vi "solar_voy_def Export (Mods_Limits).vi"(10 "CMD":enum8{"CMD", "TLM"}(ring), 11 "LIMITS":T1) -> (3 "LIMITS_DEF":string)   [LabVIEW 2018]
doc: "This exports a COSMOS limits modifier to string."
uses:
  solar_voy_def_ctl MODIFIERS LIMITS.ctl
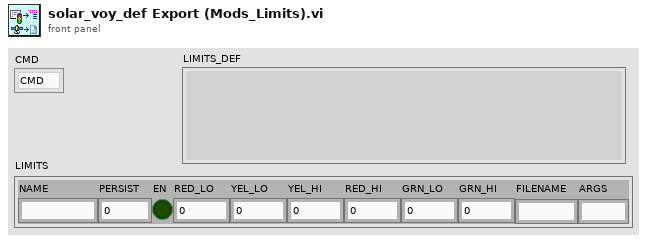
[diagram p1: front panel]
types:
  T1 = typedef "solar_voy_def_ctl MODIFIERS LIMITS.ctl" = cluster{"NAME":string, "PERSIST":i32, "EN":bool, "RED_LO":dbl, "YEL_LO":dbl, "YEL_HI":dbl, "RED_HI":dbl, "GRN_LO":dbl, "GRN_HI":dbl, "FILENAME":string, "ARGS":string}
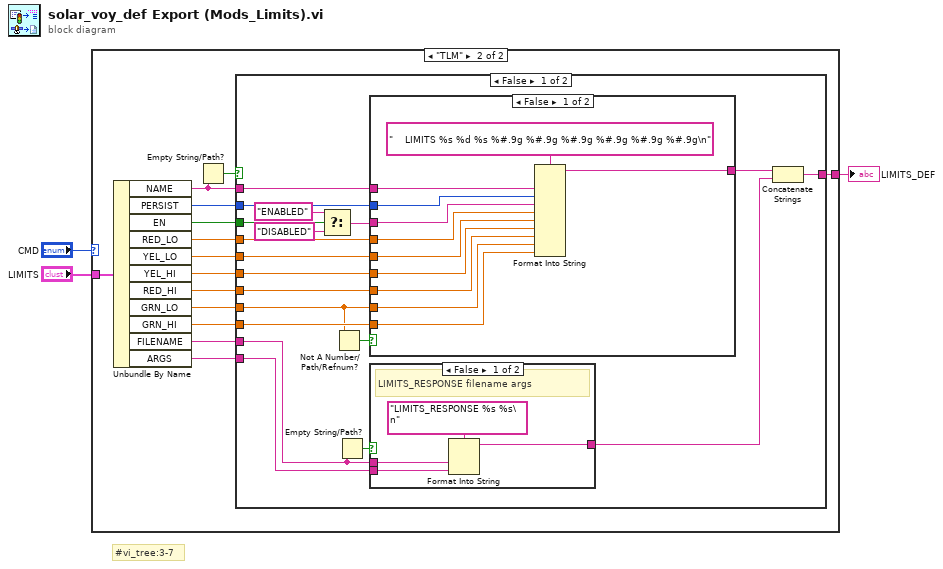
[diagram p0: block diagram]
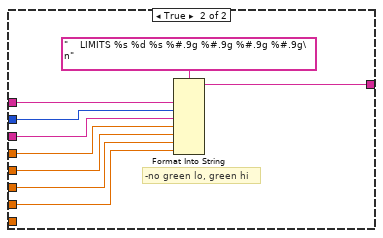
[diagram p4: hidden frame]
diagram:
  # "#vi_tree:3-7"
  n1 = case shown="\"TLM\"" "CMD" {
    tunnel: "LIMITS" -> [_ w17]
    tunnel: [_ w7] -> w1
    frame "CMD" {
      # "Commands have no limits"
    }
    frame "TLM" {
      n2 = Unbundle By Name(w17) -> ("NAME"=w5:string, "PERSIST"=w16:i32, "EN"=w15:bool, "RED_LO"=w14:dbl, "YEL_LO"=w13:dbl, "YEL_HI"=w12:dbl, "RED_HI"=w11:dbl, "GRN_LO"=w9:dbl, "GRN_HI"=w10:dbl, "FILENAME"=w8:string, "ARGS"=w6:string)
      n3 = Empty String/Path?(string/path=w5) -> (empty?=w4:bool)
      n4 = case shown="False" w4 {
        tunnel: w5 -> [w36 _]
        tunnel: w16 -> [w35 _]
        tunnel: w15 -> [w34 _]
        tunnel: w14 -> [w33 _]
        tunnel: w13 -> [w32 _]
        tunnel: w12 -> [w31 _]
        tunnel: w11 -> [w30 _]
        tunnel: w10 -> [w29 _]
        tunnel: w9 -> [w27 _]
        tunnel: w8 -> [w21 _]
        tunnel: [w20 _] -> w7
        tunnel: w6 -> [w18 _]
        frame False {
          n5 = Select(t="ENABLED", s=w34, f="DISABLED") -> (s? t:f=w25:string)
          n6 = Not A Number/Path/Refnum?(number/path/refnum=w27) -> (NaN/Path/Refnum?=w26:bool)
          n7 = Empty String/Path?(string/path=w21) -> (empty?=w22:bool)
          n8 = case shown="False" w26 {
            tunnel: w36 -> [w51 w60]
            tunnel: w35 -> [w50 w59]
            tunnel: w25 -> [w49 w58]
            tunnel: w33 -> [w48 w57]
            tunnel: w32 -> [w47 w56]
            tunnel: w31 -> [w46 w55]
            tunnel: w30 -> [w45 w54]
            tunnel: w27 -> [w43 _]
            tunnel: w29 -> [w42 _]
            tunnel: [w41 w52] -> w28
            frame False {
              n9 = Format Into String(format string="    LIMITS %s %d %s %#.9g %#.9g %#.9g %#.9g %#.9g %#.9g\n", w51, w50, w49, w48, w47, w46, w45, w43, w42) -> (resulting string=w41:string)  [unwired: 2 in, 1 out]
            }
            frame True {
              # "-no green lo, green hi"
              n10 = Format Into String(format string="    LIMITS %s %d %s %#.9g %#.9g %#.9g %#.9g\n", w60, w59, w58, w57, w56, w55, w54) -> (resulting string=w52:string)  [unwired: 2 in, 1 out]
            }
          }
          n11 = case shown="False" w22 {
            tunnel: w21 -> [w39 _]
            tunnel: [w38 _] -> w19
            tunnel: w18 -> [w37 _]
            frame False {
              # "LIMITS_RESPONSE filename args"
              n12 = Format Into String(format string="LIMITS_RESPONSE %s %s\n", w39, w37) -> (resulting string=w38:string)  [unwired: 2 in, 1 out]
            }
            frame True {
            }
          }
          n13 = Concatenate Strings(w28, w19) -> (w20:string)
        }
        frame True {
          # "Invalid limits name"
        }
      }
    }
  }
  "LIMITS_DEF" <- w1
